vi "CONST820目标压力测量.vi"(3 "error in (no error) 2":errorcluster caption="错误输入（无错误）", 5 "VISA resource name":refnum<visa-resource-name> caption="VISA资源名称") -> (0 "错误输出":errorcluster, 1 "目标压力值":string, 2 "VISA资源名称输出":refnum<visa-resource-name>)   [LabVIEW 2017]
panel:
  in  "等待时间（毫秒）":u32=100
  in  "写":bool=TRUE
  in  "写入缓冲区":string="MEASure:PRESsure1?"
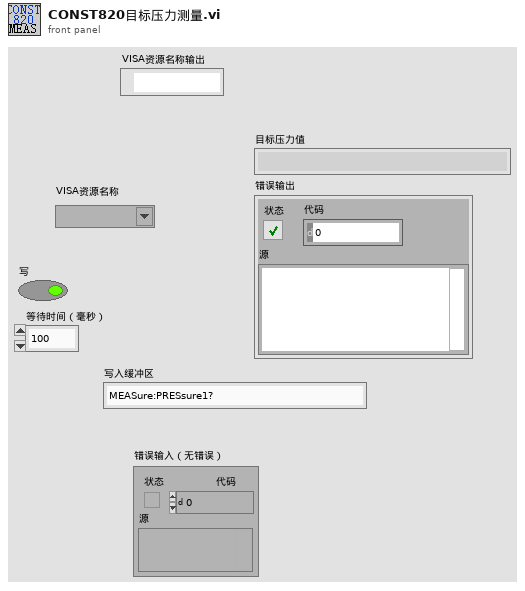
[diagram p1: front panel]
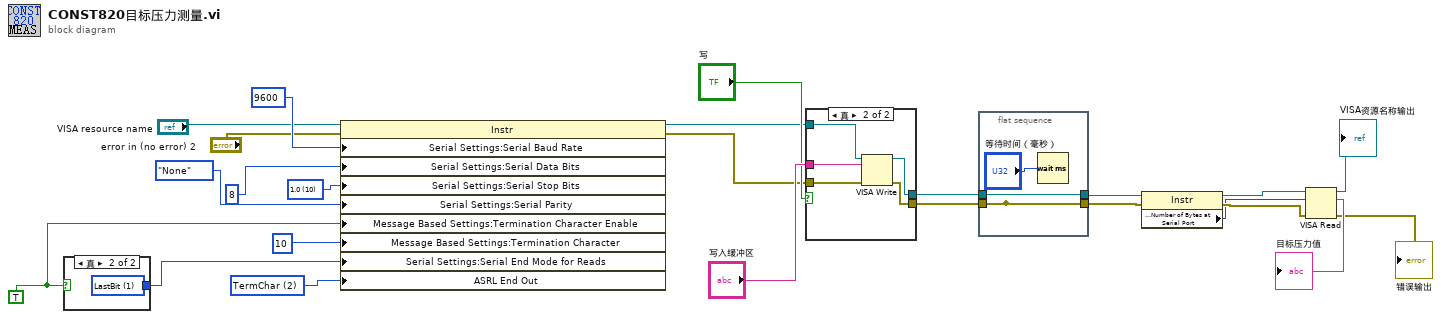
[diagram p0: block diagram]
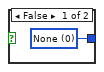
[diagram p2: hidden frame]
diagram:
  w6 = TRUE ("Enable Termination\nChar (T) 2")
  w5 = u16 2 items=["None", "Last Bit", "TermChar", "Break"] ("Serial Settings:End Mode for Writes")
  w8 = u16 10 items=["1.0"=10, "1.5"=15, "2.0"=20] ("stop bits (10: 1 bit)")
  n1 = case shown="真" w6 {
    tunnel: [w25 w26] -> w7
    frame False {
      w25 = u16 0 items=["None", "LastBit", "TermChar"] ("Serial Settings:Serial End Mode for Reads")
    }
    frame True {
      w26 = u16 1 items=["None", "LastBit", "TermChar"] ("Serial Settings:Serial End Mode for Reads")
    }
  }
  n2 = property class="Instr"(reference="VISA resource name", error in="error in (no error) 2", "Serial Settings:Serial Baud Rate"=u32 9600 ("baud rate (9600)"), "Serial Settings:Serial Data Bits"=u16 8 ("data bits (8)"), "Serial Settings:Serial Stop Bits"=w8, "Serial Settings:Serial Parity"=enum16{"None", "Odd", "Even", "Mark", "Space"}."None" ("parity (0:none)"), "Message Based Settings:Termination Character Enable"=w6, "Message Based Settings:Termination Character"=u8 10 ("termination char\n(0xA = '\\n' = LF)"), "Serial Settings:Serial End Mode for Reads"=w7, "ASRL End Out"=w5) -> (reference out=w4:refnum<visa-resource-name>, error out=w3:errorcluster)
  n3 = case shown="真" "写" {
    tunnel: "写入缓冲区" -> [_ w33]
    tunnel: [w28 w32] -> w22
    tunnel: [w27 w31] -> w21
    tunnel: w4 -> [w27 w30]
    tunnel: w3 -> [w28 w29]
    frame False {
    }
    frame True {
      n4 = VISA Write(VISA resource name=w30, write buffer=w33, error in (no error)=w29) -> (VISA resource name out=w31:refnum<visa-resource-name>, error out=w32:errorcluster)  [unwired: 1 out]
    }
  }
  n5 = flat-sequence {
    tunnel: [w34] -> _
    tunnel: w22 -> [w34]
    tunnel: w21 -> [w35]
    tunnel: [w35] -> w18
    tunnel: [w34] -> w17
    frame #0 {
      n6 = Wait (ms)(milliseconds to wait="等待时间（毫秒）") -> ()  [unwired: 1 out]
    }
  }
  n7 = property class="Instr"(reference=w18, error in=w17) -> (reference out=w20:refnum<visa-resource-name>, error out=w19:errorcluster, "Serial Settings:Number of Bytes at Serial Port"=w16:u32)
  n8 = VISA Read(VISA resource name=w20, byte count=w16, error in (no error)=w19) -> (VISA resource name out=→"VISA资源名称输出":refnum<visa-resource-name>, read buffer=→"目标压力值":string, error out=→"错误输出":errorcluster)  [unwired: 1 out]
